vi "Pacemaker ASIC Test_Save_SN Globals.vi"() -> ()   [LabVIEW 2016]
panel:
  in  "Save_SN":path
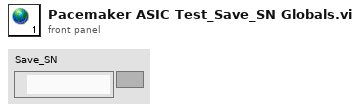
[diagram p1: front panel]
diagram:
